vi "Orange--constant.vi"() -> ()   [LabVIEW 2018]
panel:
  out "Color":u32(colorbox)
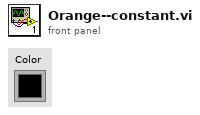
[diagram p1: front panel]
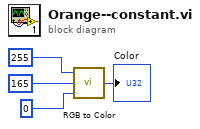
[diagram p0: block diagram]
diagram:
  n1 = call <vilib>:"RGB to Color.vi"("B"=u8 0, "G"=u8 165, "R"=u8 255) -> ("Color"=→"Color":u32)
